vi "Write ColumnNameEqualsValueFormat.vi"(8 "error in (no error)":errorcluster, 10 "ColumnNameEqualsValueFormat":string, 11 "DbConnection in":refnum<class "DbConnection.lvclass">) -> (0 "error out":errorcluster, 3 "DbConnection out":refnum<class "DbConnection.lvclass">)   [LabVIEW 2020, in "ORM.lvlib" / "DbConnection.lvclass"]
uses:
  DbConnection.lvclass
  DbConnection.lvclass/DbConnection.ctl
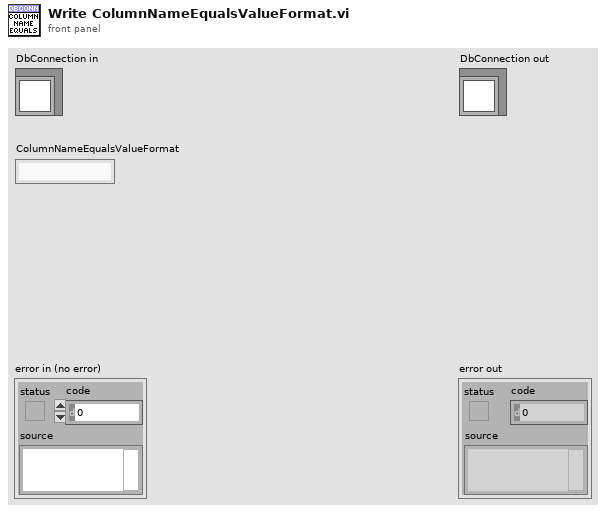
[diagram p1: front panel]
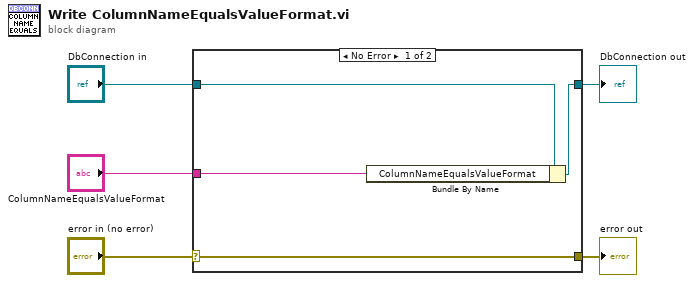
[diagram p0: block diagram]
diagram:
  n1 = case shown="No Error" "error in (no error)" {
    selector: "error in (no error)" -> [w9 w10]
    tunnel: [w9 w10] -> w4
    tunnel: [w7 w11] -> w2
    tunnel: "DbConnection in" -> [w8 w11]
    tunnel: "ColumnNameEqualsValueFormat" -> [w6 _]
    frame No Error {
      n2 = Bundle By Name(cluster=w8, "ColumnNameEqualsValueFormat"=w6) -> (w7:refnum<class "DbConnection.lvclass">)
    }
    frame Error {
    }
  }
  "error out" <- w4
  "DbConnection out" <- w2
